vi "多面板.vi"() -> ()   [LabVIEW 2014]
doc: "本范例演示了如何在子面板中查看VI。"
panel:
  in  "显示VI":u16(ring) items=["正弦波", "随机数据图", "当前时间"]
  in  "停止":bool
  # "概述：演示子面板控件如何显示不同的VI前面板。\n操作步骤：\n1. 运行VI。\n2. 选择不同的显示VI在子面板控件中显示。\n3. 单击停止，停止VI。"
  # "选中VI的属性决定子面板控件的显示方式。例如，该例中的所有VI都禁用了滚动条。所以，子面板控件上也不显示滚动条。"
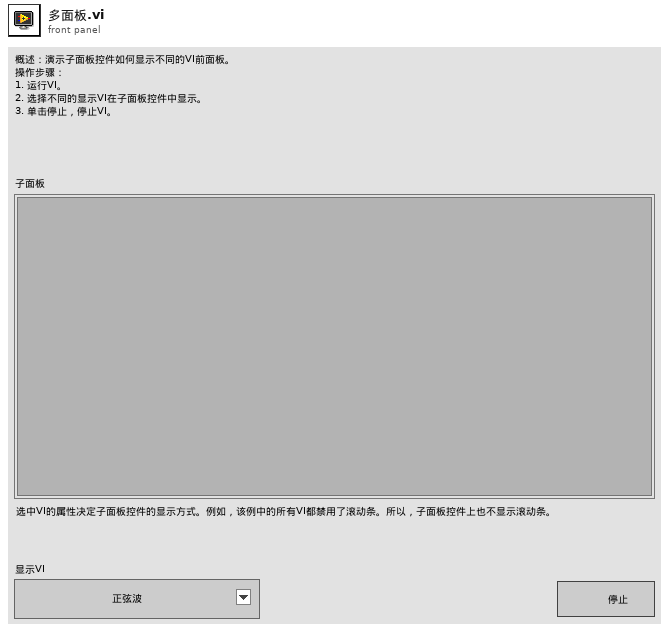
[diagram p1: front panel]
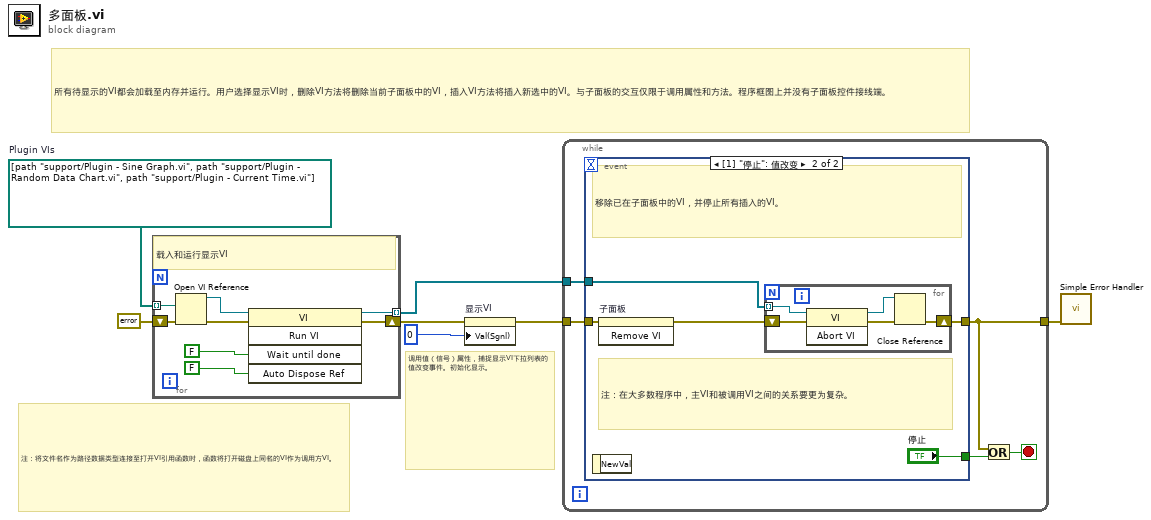
[diagram p0: block diagram]
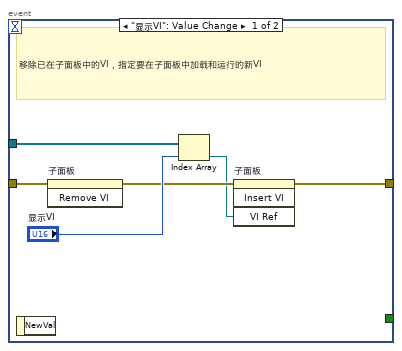
[diagram p2: hidden frame]
diagram:
  w4 = path[] [path "support/Plugin - Sine Graph.vi", path "support/Plugin - Random Data Chart.vi", path "support/Plugin - Current Time.vi"]  # Plugin VIs
  # "所有待显示的VI都会加载至内存并运行。用户选择显示VI时，删除VI方法将删除当前子面板中的VI，插入VI方法将插入新选中的VI。与子面板的交互仅限于调用属性和方法。程序框图上并没有子面板控件接线端。"
  # "注：将文件名作为路径数据类型连接至打开VI引用函数时，函数将打开磁盘上同名的VI作为调用方VI。"
  # "调用值（信号）属性，捕捉显示VI下拉列表的值改变事件。初始化显示。"
  n1 = for {
    tunnel: w4 -> [w11] mode=indexing
    tunnel: [w10] -> w1 mode=indexing
    shift-right: [w8] -> w2
    shift-left: errorcluster {"status"=FALSE, "code"=0, "source"=""} ("error constant") -> [w9]
    # "载入和运行显示VI"
    n2 = Open VI Reference(vi path=w11, error in (no error)=w9) -> (vi reference=w12:refnum<vi>, error out=w13:errorcluster)  [unwired: 4 in]
    n3 = invoke class="VI" method="Run VI"(reference=w12, error in=w13, "Wait until done"=FALSE ("Wait Until Done"), "Auto Dispose Ref"=FALSE ("Auto Dispose Reference")) -> (reference out=w10:refnum<vi>, error out=w8:errorcluster)  [unwired: 1 in, 3 out]
  }
  n4 = property on="显示VI" class="下拉列表 (严格)"(error in=w2, "Val(Sgnl)"=u16 0 ("Value (Signaling)")) -> (error out=w7:errorcluster)  [unwired: 1 in, 1 out]
  n5 = while {
    tunnel: w7 -> [w16]
    tunnel: [w18] -> w5
    tunnel: w1 -> [w17]
    stop <- w19 stop-if-true
    n6 = event shown="[1] \"停止\": 值改变" {
      selector: _ -> [_ _]
      dyn-events: _ -> [_ _]
      timeout: _ -> [_ _]
      tunnel: [_ "停止"] -> w20
      tunnel: [w25 w28] -> w18
      tunnel: w17 -> [w24 w29]
      tunnel: w16 -> [w21 w27]
      event "显示VI": Value Change {
        # "移除已在子面板中的VI，指定要在子面板中加载和运行的新VI"
        n7 = event-data() -> ()  [unwired: 1 in, 1 out]
        n8 = invoke on="子面板" class="SubPnl" method="Remove VI"(error in=w21) -> (error out=w23:errorcluster)  [unwired: 2 in, 2 out]
        n9 = Index Array(array=w24, index="显示VI") -> (element=w22:refnum<vi>)
        n10 = invoke on="子面板" class="SubPanel" method="Insert VI"(error in=w23, "VI Ref"=w22) -> (error out=w25:errorcluster)  [unwired: 2 in, 3 out]
      }
      event "停止": Value Change {
        # "注：在大多数程序中，主VI和被调用VI之间的关系要更为复杂。"
        # "移除已在子面板中的VI，并停止所有插入的VI。"
        n11 = event-data() -> ()  [unwired: 1 in, 1 out]
        n12 = invoke on="子面板" class="SubPnl" method="Remove VI"(error in=w27) -> (error out=w30:errorcluster)  [unwired: 2 in, 2 out]
        n13 = for {
          shift-right: [w32] -> w28
          shift-left: w30 -> [w36]
          tunnel: w29 -> [w35] mode=indexing
          n14 = invoke class="VI" method="Abort VI"(reference=w35, error in=w36) -> (reference out=w33:refnum<vi>, error out=w34:errorcluster)  [unwired: 1 in, 1 out]
          n15 = Close Reference(reference=w33, error in (no error)=w34) -> (error out=w32:errorcluster)
        }
      }
    }
    n16 = Or(x=w18, y=w20) -> (x .or. y?=w19:bool)
  }
  n17 = call <vilib>:"Simple Error Handler.vi"("error in (no error)"=w5) -> ()  [unwired: 4 in, 5 out]
